vi "Teleop.vi"(0 "Call Context":T2, 1 "Match Info":T1={"Autonomous Elapsed Seconds"=0.0, "TeleOp Elapsed Seconds"=0.0, "Disabled Elapsed Seconds"=0.0, "Visited Autonomous"=FALSE, "Visited TeleOp"=FALSE, "Visited Disabled"=FALSE, "Autonomous Settings"={"Autonomous Style"=enum."Independent", "VI Refnum"=refnum}}) -> ()   [LabVIEW 2013]
doc: "This VI is called for each TeleOp packet received from the DS where the robot is not disabled. It is often used to read from the joysticks and update I/O or to update setpoints for timed control loops. It should complete and return within 20 milliseconds or it may miss DS packets."
uses:
  <vilib>/Rock Robotics/WPI/DriverStation/WPI_DriverStationDerivedRobotMode.ctl
  <vilib>/Rock Robotics/WPI/DriverStation/WPI_DriverStationMatch Info.ctl
  <vilib>/Rock Robotics/WPI/Solenoid/WPI_SolenoidValue.ctl
  Robot Global Data.vi
  <vilib>/Rock Robotics/WPI/Solenoid/Deprecated/WPI_SolenoidGetBool.vi
  <vilib>/Rock Robotics/WPI/Solenoid/WPI_SolenoidSetEnum.vi
  <vilib>/Rock Robotics/WPI/Joystick/WPI_JoystickGetSetRefNum.vi
  <vilib>/Rock Robotics/WPI/RobotDrive/WPI_RobotDriveGetSetRefNum.vi
panel:
  out "Voltage":dbl
  out "Value":bool
  out "Boolean 2":bool
  out "Boolean 1":bool
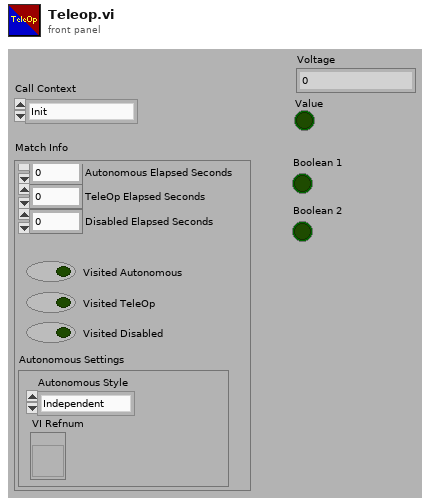
[diagram p1: front panel]
types:
  T1 = typedef "WPI_DriverStationMatch Info.ctl" = cluster{"Autonomous Elapsed Seconds":dbl, "TeleOp Elapsed Seconds":dbl, "Disabled Elapsed Seconds":dbl, "Visited Autonomous":bool, "Visited TeleOp":bool, "Visited Disabled":bool, "Autonomous Settings":cluster{"Autonomous Style":enum16{"Iterative", "Independent"}, "VI Refnum":refnum<vi>}}
  T2 = typedef "WPI_DriverStationDerivedRobotMode.ctl" = enum16{"Init", "Execute", "Stop"}
  T3 = typedef "WPI_AnalogChannelDevRef.ctl" = cluster{"DevStatus":errorcluster, "Analog Module":T4, "Analog Channel":T5}
  T4 = typedef "FPGA_TypedefAnalogModule.ctl" = enum16{"Analog Module 1", "Analog Module 2"}
  T5 = typedef "FPGA_AIChannel.ctl" = enum8{"AI 1", "AI 2", "AI 3", "AI 4", "AI 5", "AI 6", "AI 7", "AI 8", "Invalid"}
  T6 = typedef "WPI_JoystickDevRef.ctl" = cluster{"Device":T7}
  T7 = typedef "WPI_JoystickDeviceEnum.ctl" = enum16{"USB 1", "USB 2", "USB 3", "USB 4", "Kinect 1", "Kinect 2"}
  T8 = typedef "WPI_JoystickButtonState.ctl" = cluster{"Button 1":bool, "Button 2":bool, "Button 3":bool, "Button 4":bool, "Button 5":bool, "Button 6":bool, "Button 7":bool, "Button 8":bool, "Button 9":bool, "Button 10":bool, "Button 11":bool, "Button 12":bool}
  T9 = cluster{"axis 1 (x)":dbl, "axis 2 (y)":dbl, "axis 3 (throttle)":dbl, "axis 4":dbl, "axis 5":dbl, "axis 6":dbl}
  T10 = typedef "WPI_RelayDevRef.ctl" = cluster{"DevStatus":errorcluster, "Relay Channel":T11, "Digital Module":T12, "Relay Direction":T13}
  T11 = typedef "FPGA_DIORelayChannel.ctl" = enum8{"Relay 1", "Relay 2", "Relay 3", "Relay 4", "Relay 5", "Relay 6", "Relay 7", "Relay 8", "Invalid"}
  T12 = typedef "FPGA_TypedefDigitalModule.ctl" = enum16{"Digital Module 1", "Digital Module 2"}
  T13 = typedef "WPI_RelayDirection.ctl" = enum16{"Both directions", "Forward only", "Reverse only"}
  T14 = typedef "WPI_RobotDriveDevRef.ctl" = cluster{"DevStatus":errorcluster, "Motors[]":T15[], "Square Inputs":bool, "Max Output":dbl, "Isochronous":bool}
  T15 = typedef "WPI_MotorControlDeviceRef.ctl" = cluster{"DeviceStatus":errorcluster, "Type":enum16{"PWM", "CAN"}, "PWM":cluster{"Digital Module":T12, "PWM Channel":T16, "DeadBand":T17}, "CAN":cluster{"Device Number":u8, "Control Mode":T18, "Semaphore":T19, "Max Vout":dbl}, "Invert":bool, "TransformRef":T20, "InvTransformRef":T20}
  T16 = typedef "FPGA_DIOPWMChannel.ctl" = enum8{"PWM 1", "PWM 2", "PWM 3", "PWM 4", "PWM 5", "PWM 6", "PWM 7", "PWM 8", "PWM 9", "PWM 10", "Invalid"}
  T17 = typedef "WPI_PWMDeadband.ctl" = cluster{"Name":string, "maxPositivePwm":i32, "minPositivePwm":i32, "centerPwm":i32, "maxNegativePwm":i32, "minNegativePwm":i32, "angularRange":u16}
  T18 = typedef "WPI_CANJaguar_ControlMode.ctl" = enum8{"Percent VBus", "Current", "Speed", "Position", "Voltage"}
  T19 = typedef "Semaphore RefNum" = refnum<k1>
  T20 = typedef "WPI_PWMTransform_ConPane.ctl" = refnum<vi>
  T21 = typedef "WPI_DigitalInputDevRef.ctl" = cluster{"DevStatus":errorcluster, "DIO Channel":T22, "Digital Module":T12}
  T22 = typedef "FPGA_DIOChannel.ctl" = enum8{"DIO 1", "DIO 2", "DIO 3", "DIO 4", "DIO 5", "DIO 6", "DIO 7", "DIO 8", "DIO 9", "DIO 10", "DIO 11", "DIO 12", "DIO 13", "DIO 14", "Invalid"}
  T23 = typedef "WPI_SolenoidDevRef.ctl" = cluster{"DevStatus":errorcluster, "Solenoid Module":T24, "Forward Solenoid Channel":T25, "Reverse Solenoid Channel":T25}
  T24 = typedef "FPGA_TypedefSolenoidModule.ctl" = enum16{"Solenoid Module 1", "Solenoid Module 2"}
  T25 = typedef "WPI_SolenoidChannel.ctl" = enum8{"Solenoid 1", "Solenoid 2", "Solenoid 3", "Solenoid 4", "Solenoid 5", "Solenoid 6", "Solenoid 7", "Solenoid 8", "Invalid"}
  T26 = typedef "WPI_SolenoidValue.ctl" = enum16{"Off", "On", "Forward", "Reverse"}
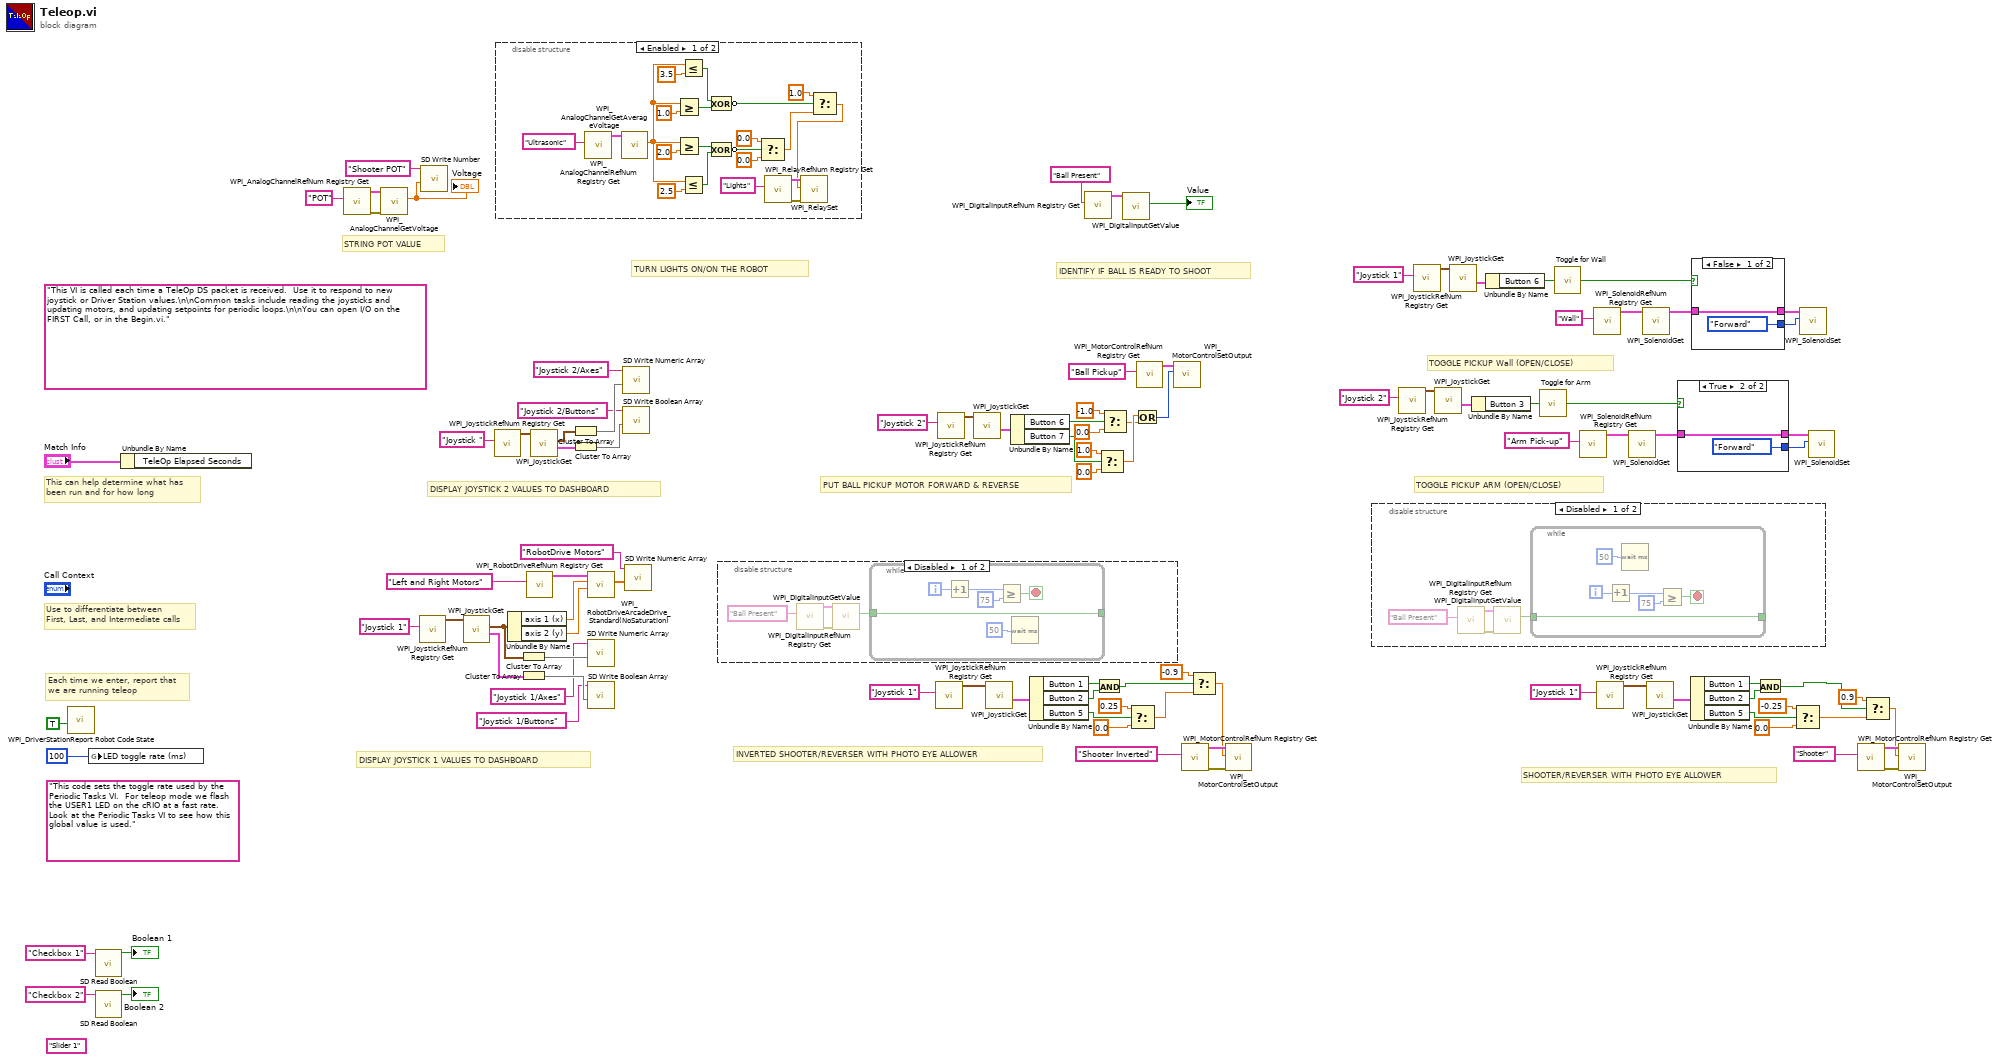
[diagram p0: block diagram]
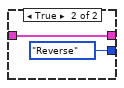
[diagram p2: hidden frame]
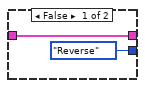
[diagram p6: hidden frame]
diagram:
  (unwired) "Slider 1" ("refnum name")
  (unwired) "This code sets the toggle rate used by the Periodic Tasks VI.  For teleop mode we flash the USER1 LED on the cRIO at a fast rate.  Look at the Periodic Tasks VI to see how this global value is used."
  (unwired) "This VI is called each time a TeleOp DS packet is received.  Use it to respond to new joystick or Driver Station values.\n\nCommon tasks include reading the joysticks and updating motors, and updating setpoints for periodic loops.\n\nYou can open I/O on the FIRST Call, or in the Begin.vi."
  # "TOGGLE PICKUP Wall (OPEN/CLOSE)"
  # "SHOOTER/REVERSER WITH PHOTO EYE ALLOWER"
  # "INVERTED SHOOTER/REVERSER WITH PHOTO EYE ALLOWER"
  # "TOGGLE PICKUP ARM (OPEN/CLOSE)"
  # "PUT BALL PICKUP MOTOR FORWARD & REVERSE"
  # "DISPLAY JOYSTICK 1 VALUES TO DASHBOARD"
  # "DISPLAY JOYSTICK 2 VALUES TO DASHBOARD"
  # "IDENTIFY IF BALL IS READY TO SHOOT"
  # "TURN LIGHTS ON/ON THE ROBOT"
  # "STRING POT VALUE"
  # "Each time we enter, report that\nwe are running teleop"
  # "Use to differentiate between\nFirst, Last, and Intermediate calls"
  # "This can help determine what has\nbeen run and for how long"
  n1 = call <vilib>:"WPI_DriverStationReport Robot Code State.vi"("TeleOp"=TRUE ("Autonomous")) -> ()  [unwired: 10 in, 1 out]
  n2 = global write "Robot Global Data.vi" "LED toggle rate (ms)"(u32 100 ("LED ms toggle rate")) -> ()
  n3 = call <vilib>:"SD Read Boolean.vi"("Name"="Checkbox 1" ("refnum name")) -> ("Boolean"=→"Boolean 1":bool)  [unwired: 8 in, 2 out]
  n4 = call <vilib>:"SD Read Boolean.vi"("Name"="Checkbox 2" ("refnum name")) -> ("Boolean"=→"Boolean 2":bool)  [unwired: 8 in, 2 out]
  n5 = Unbundle By Name("Match Info") -> ()  [unwired: 1 out]
  n6 = call <vilib>:"WPI_AnalogChannelRefNum Registry Get.vi"("refnum name"="POT") -> ("error out"=w44:errorcluster, "AIDeviceRef"=w45:T3)  [unwired: 9 in]
  n7 = call <vilib>:"WPI_AnalogChannelGetVoltage.vi"("error in (no error)"=w44, "AIDeviceRef"=w45) -> ("Voltage"=w42:dbl)  [unwired: 7 in, 2 out]
  "Voltage" <- w42
  n8 = call <vilib>:"WPI_JoystickRefNum Registry Get.vi"("refnum name"="Joystick 1") -> ("JoystickDevRef"=w95:T6)  [unwired: 1 in, 9 out]
  n9 = call <vilib>:"SD Write Number.vi"("Numeric"=w42, "Name"="Shooter POT" ("Table Prefix out")) -> ()  [unwired: 8 in, 2 out]
  n10 = call <vilib>:"WPI_JoystickGet.vi"("JoystickDevRef"=w95) -> ("Buttons"=w93:T8, "Axes"=w90:T9)  [unwired: 1 in, 4 out]
  n11 = call <vilib>:"WPI_JoystickRefNum Registry Get.vi"("refnum name"="Joystick ") -> ("JoystickDevRef"=w34:T6)  [unwired: 1 in, 9 out]
  n12 = disable-structure shown="Enabled" {
    frame Enabled {
      n13 = call <vilib>:"WPI_AnalogChannelRefNum Registry Get.vi"("refnum name"="Ultrasonic") -> ("AIDeviceRef"=w121:T3)  [unwired: 9 in, 1 out]
      n14 = call <vilib>:"WPI_AnalogChannelGetAverageVoltage.vi"("AIDeviceRef"=w121) -> ("Voltage"=w112:dbl)  [unwired: 8 in, 2 out]
      n15 = Greater Or Equal?(x=w112, y=1.0) -> (x >= y?=w115:bool)
      n16 = Greater Or Equal?(x=w112, y=2.0) -> (x >= y?=w109:bool)
      n17 = Less Or Equal?(x=w112, y=3.5) -> (x <= y?=w114:bool)
      n18 = Less Or Equal?(x=w112, y=2.5) -> (x <= y?=w110:bool)
      n19 = Compound Arithmetic op=XOR(w114, w115) -> (invert w107:bool)
      n20 = Compound Arithmetic op=XOR(w109, w110) -> (invert w108:bool)
      n21 = Select(t=0.0, s=w108, f=0.0) -> (s? t:f=w103:dbl)
      n22 = call <vilib>:"WPI_RelayRefNum Registry Get.vi"("refnum name"="Lights") -> ("error out"=w120:errorcluster, "RelayDevRef"=w119:T10)  [unwired: 9 in]
      n23 = Select(t=1.0, s=w107, f=w103) -> (s? t:f=w102:dbl)
      n24 = call <vilib>:"WPI_RelaySet.vi"("error in (no error)"=w120, "RelayValue"=w102, "RelayDevRef"=w119) -> ()  [unwired: 7 in, 2 out]
    }
    frame Disabled {
    }
  }
  n25 = Unbundle By Name(w90) -> ("axis 1 (x)"=w98:dbl, "axis 2 (y)"=w97:dbl)
  n26 = Cluster To Array(cluster=w90) -> (array=w89:dbl[])
  n27 = Cluster To Array(cluster=w93) -> (array=w92:bool[])
  n28 = call <vilib>:"WPI_RobotDriveRefNum Registry Get.vi"("refnum name"="Left and Right Motors") -> ("RobotDriveDevRef"=w99:T14)  [unwired: 1 in, 9 out]
  n29 = call <vilib>:"WPI_JoystickGet.vi"("JoystickDevRef"=w34) -> ("Buttons"=w35:T8, "Axes"=w38:T9)  [unwired: 1 in, 4 out]
  n30 = Cluster To Array(cluster=w38) -> (array=w39:dbl[])
  n31 = Cluster To Array(cluster=w35) -> (array=w36:bool[])
  n32 = call <vilib>:"WPI_RobotDriveArcadeDrive_Standard(NoSaturation).vi"("Y axis value"=w97, "X axis value"=w98, "RobotDriveDevRef"=w99) -> ("Motor Values"=w86:dbl[])  [unwired: 1 in, 7 out]
  n33 = call <vilib>:"SD Write Numeric Array.vi"("Numeric Array"=w89, "Name"="Joystick 1/Axes") -> ()  [unwired: 8 in, 2 out]
  n34 = call <vilib>:"SD Write Boolean Array.vi"("Boolean Array"=w92, "Name"="Joystick 1/Buttons") -> ()  [unwired: 8 in, 2 out]
  n35 = call <vilib>:"SD Write Numeric Array.vi"("Numeric Array"=w39, "Name"="Joystick 2/Axes") -> ()  [unwired: 8 in, 2 out]
  n36 = call <vilib>:"SD Write Boolean Array.vi"("Boolean Array"=w36, "Name"="Joystick 2/Buttons") -> ()  [unwired: 8 in, 2 out]
  n37 = call <vilib>:"SD Write Numeric Array.vi"("Numeric Array"=w86, "Name"="RobotDrive Motors") -> ()  [unwired: 8 in, 2 out]
  n38 = disable-structure shown="Disabled" {
    frame Disabled {
      n39 = call <vilib>:"WPI_DigitalInputRefNum Registry Get.vi"("refnum name"="Ball Present") -> ("error out"=w125:errorcluster, "DigitalInputDevRef"=w126:T21)  [unwired: 9 in]
      n40 = call <vilib>:"WPI_DigitalInputGetValue.vi"("error in (no error)"=w125, "DigitalInputDevRef"=w126) -> ("Value"=w127:bool)  [unwired: 7 in, 2 out]
      n41 = while {
        tunnel: [w128] -> w123
        tunnel: w127 -> [w128]
        i -> [w133]
        stop <- w130 stop-if-true
        n42 = Increment(x=w133) -> (x+1=w132:i32)
        n43 = Greater Or Equal?(x=w132, y=75) -> (x >= y?=w130:bool)
        n44 = Wait (ms)(milliseconds to wait=u32 50) -> ()  [unwired: 1 out]
      }
    }
    frame Enabled {
    }
  }
  n45 = call <vilib>:"WPI_JoystickRefNum Registry Get.vi"("refnum name"="Joystick 1") -> ("JoystickDevRef"=w74:T6)  [unwired: 9 in, 1 out]
  n46 = call <vilib>:"WPI_JoystickRefNum Registry Get.vi"("refnum name"="Joystick 2") -> ("JoystickDevRef"=w64:T6)  [unwired: 9 in, 1 out]
  n47 = call <vilib>:"WPI_JoystickGet.vi"("JoystickDevRef"=w64) -> ("Buttons"=w65:T8)  [unwired: 4 in, 2 out]
  n48 = call <vilib>:"WPI_JoystickGet.vi"("JoystickDevRef"=w74) -> ("Buttons"=w75:T8)  [unwired: 4 in, 2 out]
  n49 = Unbundle By Name(w65) -> ("Button 6"=w66:bool, "Button 7"=w62:bool)
  n50 = Unbundle By Name(w75) -> ("Button 1"=w49:bool, "Button 2"=w50:bool, "Button 5"=w27:bool)
  n51 = call <vilib>:"WPI_DigitalInputRefNum Registry Get.vi"("refnum name"="Ball Present") -> ("DigitalInputDevRef"=w31:T21)  [unwired: 9 in, 1 out]
  n52 = And(x=w49, y=w50) -> (x .and. y?=w15:bool)
  n53 = Select(t=1.0, s=w62, f=0.0) -> (s? t:f=w61:dbl)
  n54 = Select(t=-1.0, s=w66, f=0.0) -> (s? t:f=w60:dbl)
  n55 = call <vilib>:"WPI_DigitalInputGetValue.vi"("DigitalInputDevRef"=w31) -> ("Value"=→"Value":bool)  [unwired: 8 in, 2 out]
  n56 = Select(t=0.25, s=w27, f=0.0) -> (s? t:f=w26:dbl)
  n57 = Or(x=w61, y=w60) -> (x .or. y?=w59:i32)
  n58 = call <vilib>:"WPI_MotorControlRefNum Registry Get.vi"("refnum name"="Ball Pickup") -> ("MotorControlDevRef"=w71:T15)  [unwired: 9 in, 1 out]
  n59 = call <vilib>:"WPI_MotorControlSetOutput.vi"("Output"=w59, "MotorControlDevRef"=w71) -> ()  [unwired: 7 in, 3 out]
  n60 = call <vilib>:"WPI_MotorControlRefNum Registry Get.vi"("refnum name"="Shooter Inverted") -> ("error out"=w47:errorcluster, "MotorControlDevRef"=w48:T15)  [unwired: 9 in]
  n61 = Select(t=-0.9, s=w15, f=w26) -> (s? t:f=w22:dbl)
  n62 = call <vilib>:"WPI_MotorControlSetOutput.vi"("error in (no error)"=w47, "Output"=w22, "MotorControlDevRef"=w48) -> ()  [unwired: 6 in, 3 out]
  n63 = disable-structure shown="Disabled" {
    frame Disabled {
      n64 = call <vilib>:"WPI_DigitalInputRefNum Registry Get.vi"("refnum name"="Ball Present") -> ("error out"=w136:errorcluster, "DigitalInputDevRef"=w135:T21)  [unwired: 9 in]
      n65 = call <vilib>:"WPI_DigitalInputGetValue.vi"("error in (no error)"=w136, "DigitalInputDevRef"=w135) -> ("Value"=w134:bool)  [unwired: 7 in, 2 out]
      n66 = while {
        tunnel: [w138] -> _
        tunnel: w134 -> [w138]
        i -> [w143]
        stop <- w140 stop-if-true
        n67 = Increment(x=w143) -> (x+1=w142:i32)
        n68 = Wait (ms)(milliseconds to wait=u32 50) -> ()  [unwired: 1 out]
        n69 = Greater Or Equal?(x=w142, y=75) -> (x >= y?=w140:bool)
      }
    }
    frame Enabled {
    }
  }
  n70 = call <vilib>:"WPI_JoystickRefNum Registry Get.vi"("refnum name"="Joystick 2") -> ("JoystickDevRef"=w56:T6)  [unwired: 9 in, 1 out]
  n71 = call <vilib>:"WPI_JoystickRefNum Registry Get.vi"("refnum name"="Joystick 1") -> ("JoystickDevRef"=w11:T6)  [unwired: 9 in, 1 out]
  n72 = call <vilib>:"WPI_JoystickGet.vi"("JoystickDevRef"=w56) -> ("Buttons"=w55:T8)  [unwired: 4 in, 2 out]
  n73 = call <vilib>:"WPI_JoystickGet.vi"("JoystickDevRef"=w11) -> ("Buttons"=w10:T8)  [unwired: 4 in, 2 out]
  n74 = Unbundle By Name(w55) -> ("Button 3"=w1:bool)
  n75 = Unbundle By Name(w10) -> ("Button 6"=w4:bool)
  n76 = call "Toggle for Arm.vi"("Input"=w1) -> ("Toggled Output"=w2:bool)
  n77 = call "Toggle for Wall.vi"("Input"=w4) -> ("Toggled Output"=w3:bool)
  n78 = call <vilib>:"WPI_SolenoidRefNum Registry Get.vi"("refnum name"="Arm Pick-up") -> ("SolenoidDevRef"=w54:T23)  [unwired: 9 in, 1 out]
  n79 = call <vilib>:"WPI_SolenoidRefNum Registry Get.vi"("refnum name"="Wall") -> ("SolenoidDevRef"=w9:T23)  [unwired: 9 in, 1 out]
  n80 = call <vilib>:"WPI_JoystickRefNum Registry Get.vi"("refnum name"="Joystick 1") -> ("JoystickDevRef"=w80:T6)  [unwired: 9 in, 1 out]
  n81 = call-poly <vilib>:"WPI_SolenoidGet.vi"("SolenoidDevRef"=w54) -> ("SolenoidDevRef"=w53:T23)  [unwired: 8 in, 2 out]
  n82 = call-poly <vilib>:"WPI_SolenoidGet.vi"("SolenoidDevRef"=w9) -> ("SolenoidDevRef"=w6:T23)  [unwired: 8 in, 2 out]
  n83 = call <vilib>:"WPI_JoystickGet.vi"("JoystickDevRef"=w80) -> ("Buttons"=w79:T8)  [unwired: 4 in, 2 out]
  n84 = case shown="True" w2 {
    tunnel: w53 -> [w145 w147]
    tunnel: [w145 w147] -> w52
    tunnel: [WPI_SolenoidValue."Reverse" ("Value") WPI_SolenoidValue."Forward" ("Value")] -> w51
    frame False {
    }
    frame True {
    }
  }
  n85 = Unbundle By Name(w79) -> ("Button 1"=w28:bool, "Button 2"=w29:bool, "Button 5"=w21:bool)
  n86 = case shown="False" w3 {
    tunnel: w6 -> [w149 w151]
    tunnel: [w149 w151] -> w7
    tunnel: [WPI_SolenoidValue."Forward" ("Value") WPI_SolenoidValue."Reverse" ("Value")] -> w8
    frame False {
    }
    frame True {
    }
  }
  n87 = And(x=w28, y=w29) -> (x .and. y?=w14:bool)
  n88 = Select(t=-0.25, s=w21, f=0.0) -> (s? t:f=w19:dbl)
  n89 = call-poly <vilib>:"WPI_SolenoidSet.vi"("Value"=w8, "SolenoidDevRef"=w7) -> ()  [unwired: 8 in, 2 out]
  n90 = call-poly <vilib>:"WPI_SolenoidSet.vi"("Value"=w51, "SolenoidDevRef"=w52) -> ()  [unwired: 8 in, 2 out]
  n91 = call <vilib>:"WPI_MotorControlRefNum Registry Get.vi"("refnum name"="Shooter") -> ("error out"=w77:errorcluster, "MotorControlDevRef"=w76:T15)  [unwired: 9 in]
  n92 = Select(t=0.9, s=w14, f=w19) -> (s? t:f=w16:dbl)
  n93 = call <vilib>:"WPI_MotorControlSetOutput.vi"("error in (no error)"=w77, "Output"=w16, "MotorControlDevRef"=w76) -> ()  [unwired: 6 in, 3 out]
